vi "solar_voy_def Parse Args.vi"(11 "String":string) -> (3 "Arguments":string[](array[string]))   [LabVIEW 2018]
doc: "This parses the string into arguments separated by whitespace."
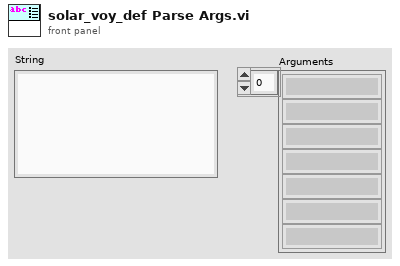
[diagram p1: front panel]
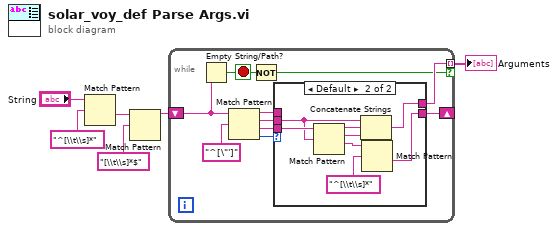
[diagram p0: block diagram]
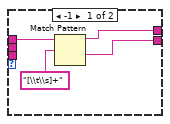
[diagram p2: hidden frame]
diagram:
  n1 = Match Pattern(string="String", regular expression="^[\\t\\s]*") -> (after substring=w5:string)  [unwired: 1 in, 3 out]
  n2 = Match Pattern(string=w5, regular expression="[\\t\\s]*$") -> (before substring=w2:string)  [unwired: 1 in, 3 out]
  n3 = while {
    shift-right: [w7] -> _
    shift-left: w2 -> [w10]
    tunnel: [w11] -> w1 mode=indexing if=w8
    stop <- w9 stop-if-true
    n4 = Empty String/Path?(string/path=w10) -> (empty?=w9:bool)
    n5 = Match Pattern(string=w10, regular expression="^[\"']") -> (before substring=w13:string, match substring=w12:string, after substring=w14:string, offset past match=w15:i32)  [unwired: 1 in]
    n6 = Not(x=w9) -> (.not. x?=w8:bool)
    n7 = case shown="Default" w15 {
      tunnel: w14 -> [_ w28]
      tunnel: w13 -> [w19 _]
      tunnel: w12 -> [_ w21]
      tunnel: [w18 w25] -> w11
      tunnel: [w17 w22] -> w7
      frame -1 {
        n8 = Match Pattern(string=w19, regular expression="[\\t\\s]+") -> (before substring=w18:string, after substring=w17:string)  [unwired: 1 in, 2 out]
      }
      frame Default {
        n9 = Match Pattern(string=w28, regular expression=w21) -> (before substring=w27:string, match substring=w26:string, after substring=w23:string)  [unwired: 1 in, 1 out]
        n10 = Concatenate Strings(w21, w27, w26) -> (w25:string)
        n11 = Match Pattern(string=w23, regular expression="^[\\t\\s]*") -> (after substring=w22:string)  [unwired: 1 in, 3 out]
      }
    }
  }
  "Arguments" <- w1
